vi "Measurements Add Items UI_Measure-Scope SP.vi"() -> ()   [LabVIEW 2012]
uses:
  Measurement Add Itmes Operations_Mesa.ctl
  <vilib>/Utility/miscctls.llb/LVPositionTypeDef.ctl
  Measure Operations_Meas.ctl
  Data Structure.llb/Function Variable Parameter Operations-Scope SP.ctl
  Data Structure.llb/Sub Panel Status Flag_DStr-Scope SP.vi
panel:
  out "Tab":enum32{"Volt", "Percent"}(tab)
  in  "Level":cluster{"High":dbl, "Mid":dbl, "Low":dbl} {"Low" min=-20.0 max=20.0 step=0.01 scale=-20.0..20.0; "Mid" min=-20.0 max=20.0 step=0.01 scale=-20.0..20.0 scale format="%#.2g"; "High" min=-20.0 max=20.0 step=0.01 scale=-20.0..20.0 scale format="%#.2f"}
  in  "Perc":cluster{"High":dbl, "Mid":dbl, "Low":dbl} {"Low" min=0.0 max=100.0 step=0.01 scale=0.0..100.0; "Mid" min=0.0 max=100.0 step=0.01 scale=0.0..100.0 scale format="%#.2g"; "High" min=0.0 max=100.0 step=0.01 scale=0.0..100.0 scale format="%#.2f"}
  in  "Config":T1
  in  "Temp":T3={"message"=variant, "measure"=refnum, "error"={"status"=FALSE, "code"=0, "source"=""}, "LevelRange"={"Max"=0.0, "Min"=0.0}, "Para"=1, "Percent"={"High"=0.0, "Mid"=0.0, "Low"=0.0}, "Level"={"High"=0.0, "Mid"=0.0, "Low"=0.0}}
  in  "Percent":i32(ring)=2 caption="百分比方式" items=["高低", "大小", "谷峰"]
  in  "Unit":i32(ring)=1 caption="单位" items=["伏特", "百分比"]
  in  "Help":bool
  in  "More...":bool
  in  "Cancel":bool
  in  "OK":bool
  in  "OtherChan":i32(ring) caption="其他通道" items=["0", "1"]
  in  "ParaSelec":i32(ring)=1 caption="测量参数" items=["设置参考电平", "频率", "平均频率", "FFT 频率", "周期", "平均周期", "上升时间", "下降时间", "上升压摆率", "下降压摆率", "过冲量", "预冲", "电压均方根", "电压周期均方根", "交流估计", "FFT幅值", "电压均值", "电压周期均值 ", "直流估计", "电压最大值", "电压最小值", "电压峰峰值", "电压高值", "电压低值 ", "电压幅值", "电压极点", "电压谷点", "电压最大差点", "负带宽", "正带宽", "负占空比", "正占空比", "积分", "面积", "周期面积", "延时", "相位延时", "低参考电压", "中参考电压", "高参考电压"]
  in  "Chan":i32(ring) caption="选择通道" items=["0", "1"]
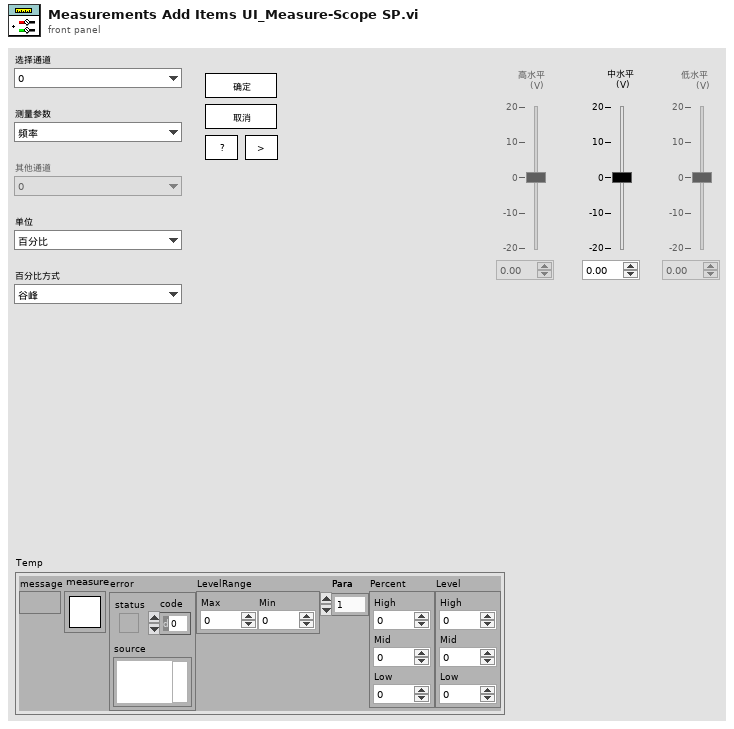
[diagram p1: front panel]
types:
  T1 = cluster{"Chan0":i32, "Para":string, "Chan1":i32, "Unit":i32, "Percent":i32, "High":dbl, "Mid":dbl, "Low":dbl, "ParaIndex":i32}
  T2 = typedef "Queue RefNum" = refnum<k1>
  T3 = cluster{"message":variant, "measure":T2, "error":errorcluster, "LevelRange":cluster{"Max":dbl, "Min":dbl}, "Para":i32, "Percent":cluster{"High":dbl, "Mid":dbl, "Low":dbl}, "Level":cluster{"High":dbl, "Mid":dbl, "Low":dbl}}
  T4 = typedef "Measurement Add Itmes Operations_Mesa.ctl" = enum16{"Initialize", "Initialize FP", "Idle", "Refresh FP", "ErrorHandle", "Close", "Exit"}
  T5 = typedef "LVPositionTypeDef.ctl" = cluster{"Left":i32, "Top":i32}
  T6 = typedef "LVRectTypeDef.ctl" = cluster{"Left":i16, "Top":i16, "Right":i16, "Bottom":i16}
  T7 = typedef "Function Variable Parameter Operations-Scope SP.ctl" = enum16{"Set", "Get"}
  T8 = typedef "Measure Operations_Meas.ctl" = enum16{"Add", "Config&Read", "Delete", "Clear"}
  T9 = cluster{"Para.":cluster{"Chans":cluster{"String":string, "Value":ext}[], "LevelRange":cluster{"Max":dbl, "Min":dbl}, "InstruHandle":refnum<k15>}, "Value":cluster{"Chan0":i32, "Para":string, "Chan1":i32, "Unit":i32, "Percent":i32, "High":dbl, "Mid":dbl, "Low":dbl, "ParaIndex":i32}[]}
  T10 = typedef "System Paths_FS-Scope SP.ctl" = cluster{"DeviceInfo":path, "SystemConstant":path, "INIDir":path}
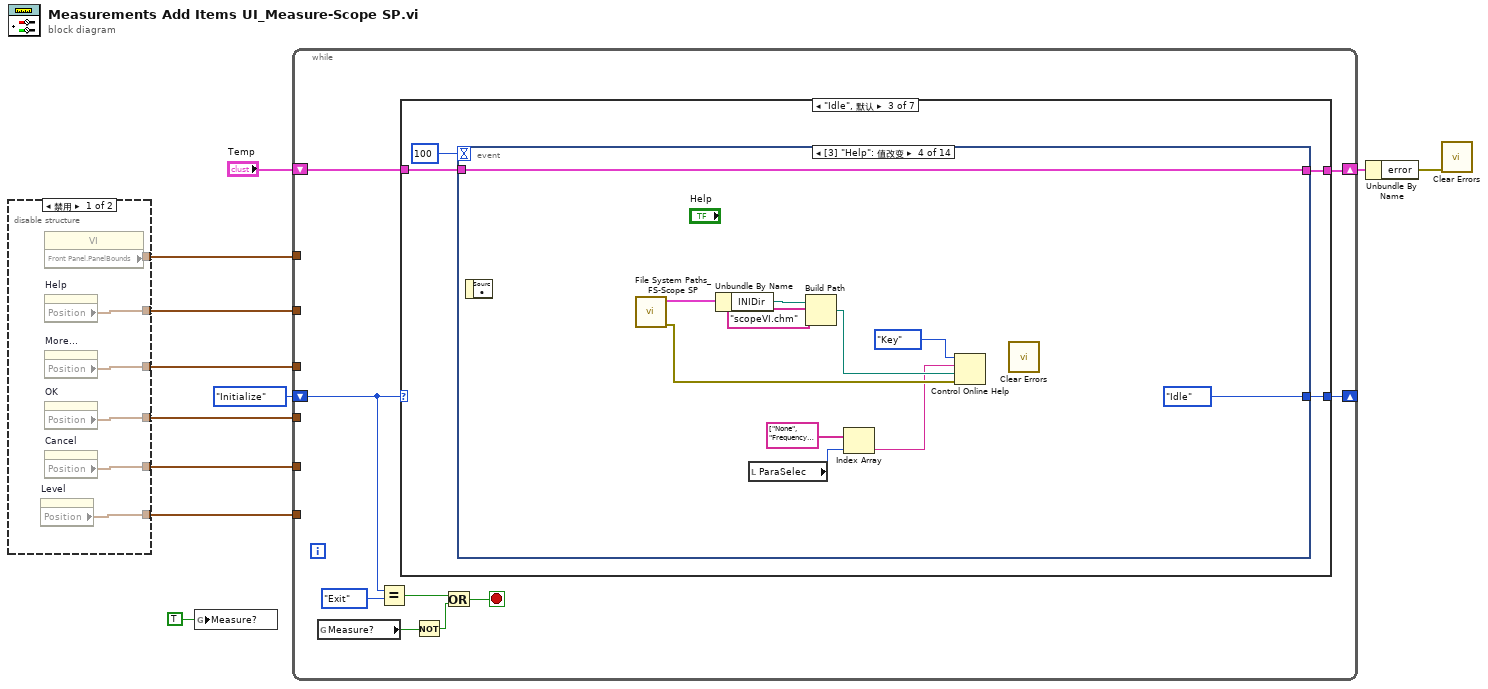
[diagram p0: block diagram]
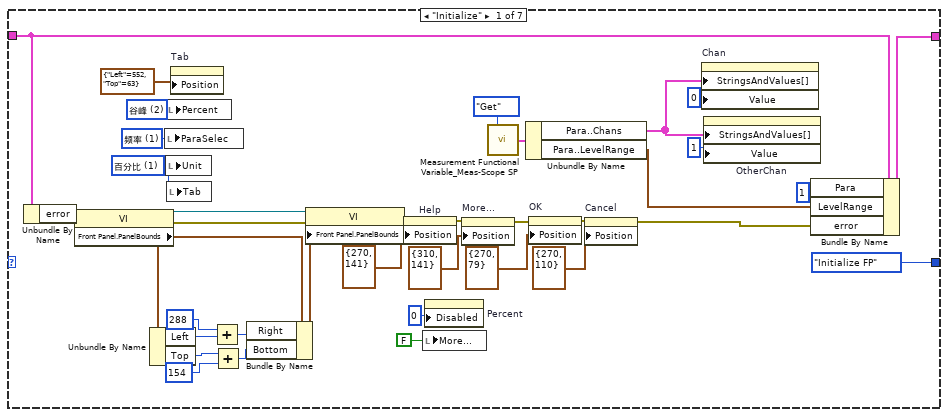
[diagram p3: hidden frame]
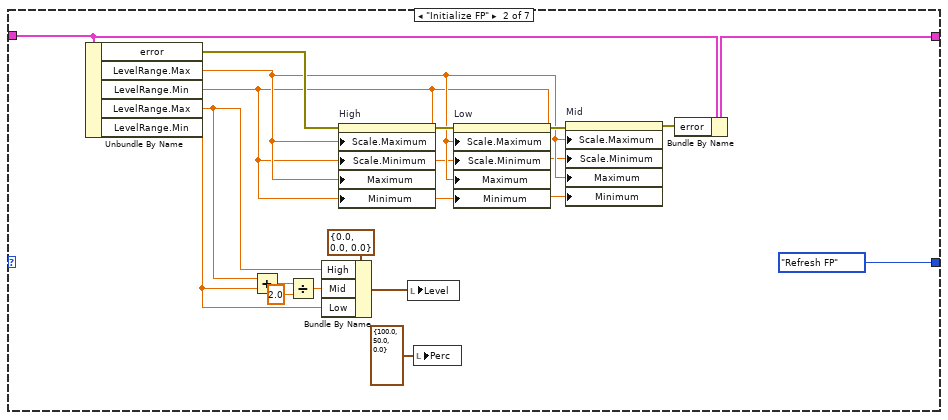
[diagram p4: hidden frame]
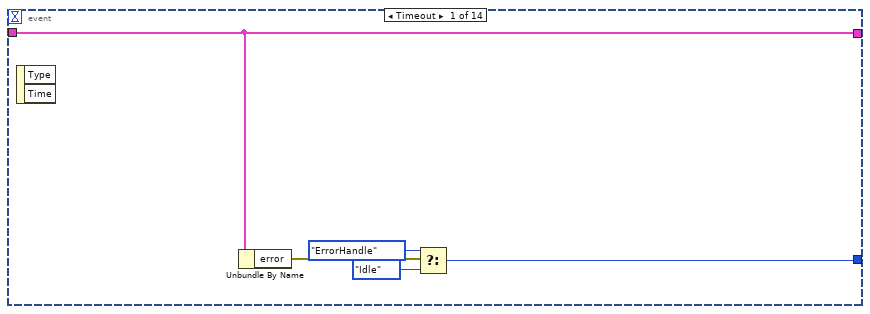
[diagram p5: hidden frame]
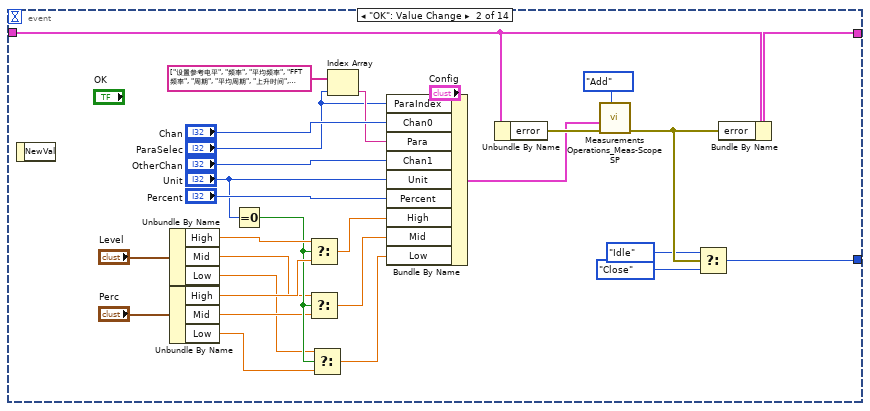
[diagram p6: hidden frame]
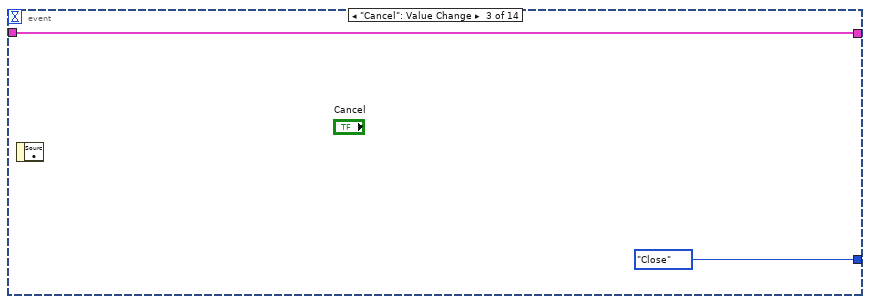
[diagram p7: hidden frame]
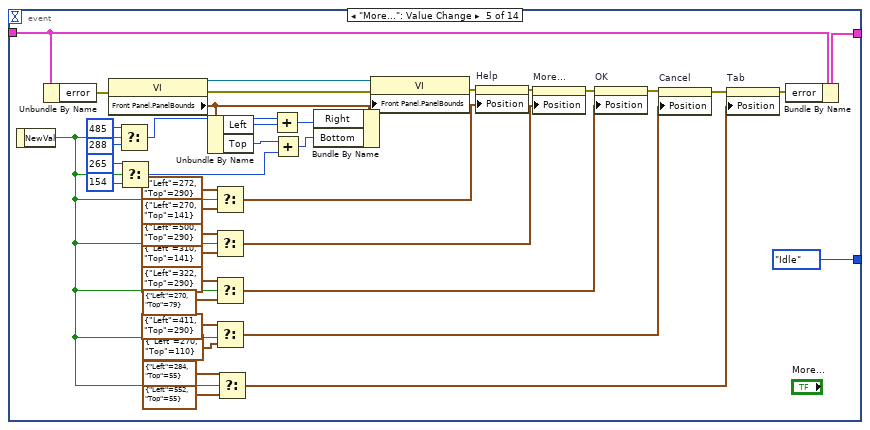
[diagram p8: hidden frame]
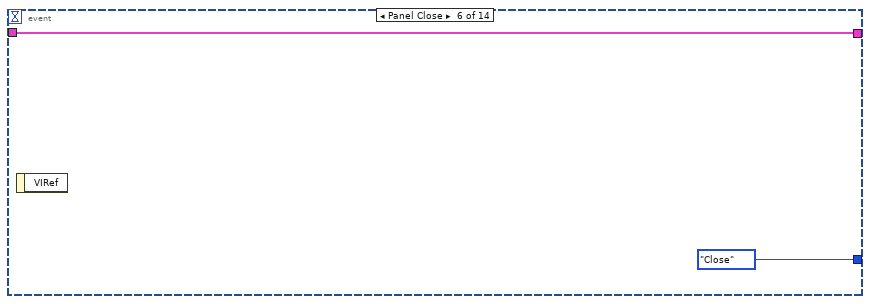
[diagram p9: hidden frame]
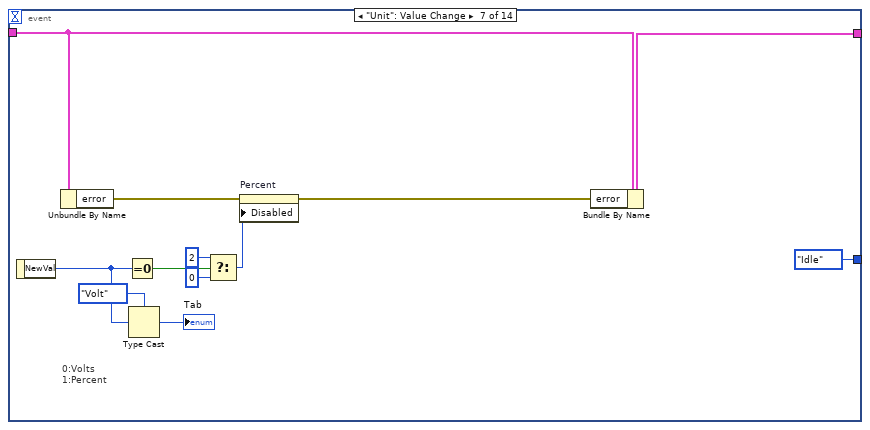
[diagram p10: hidden frame]
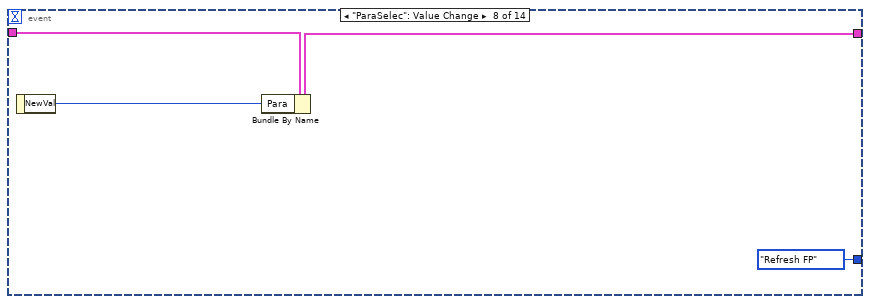
[diagram p11: hidden frame]
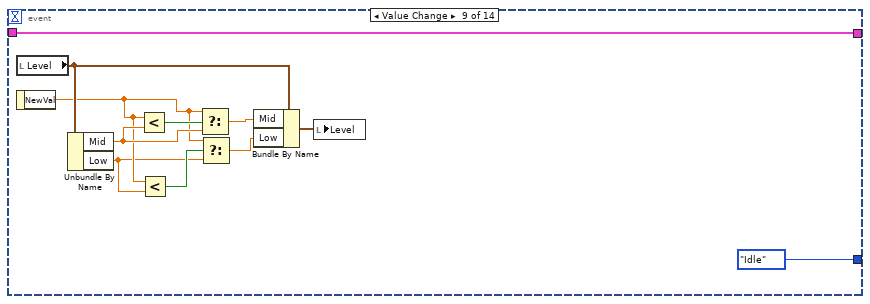
[diagram p12: hidden frame]
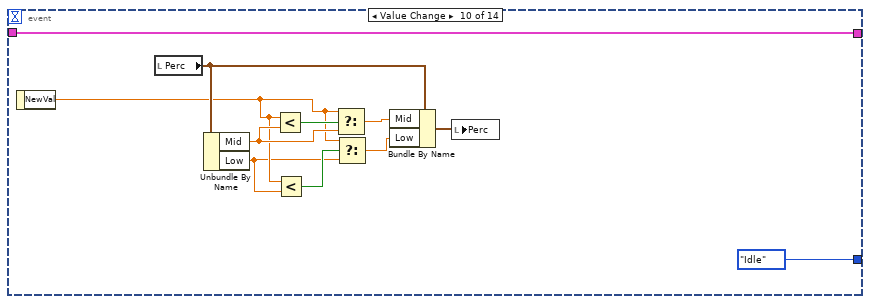
[diagram p13: hidden frame]
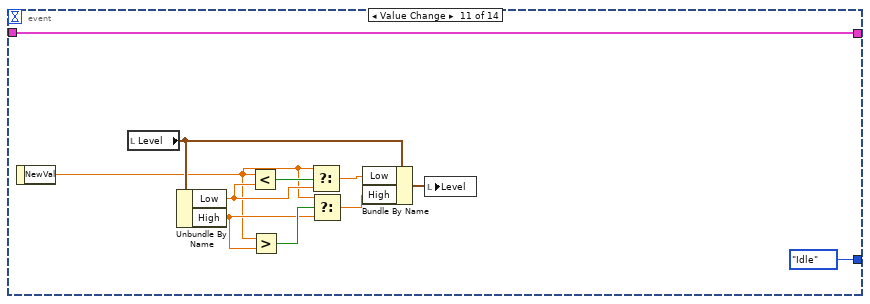
[diagram p14: hidden frame]
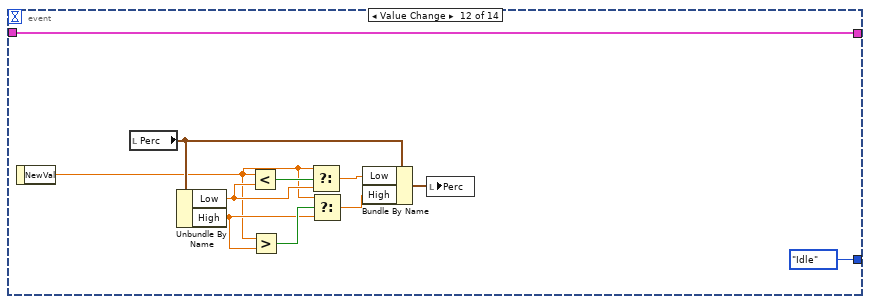
[diagram p15: hidden frame]
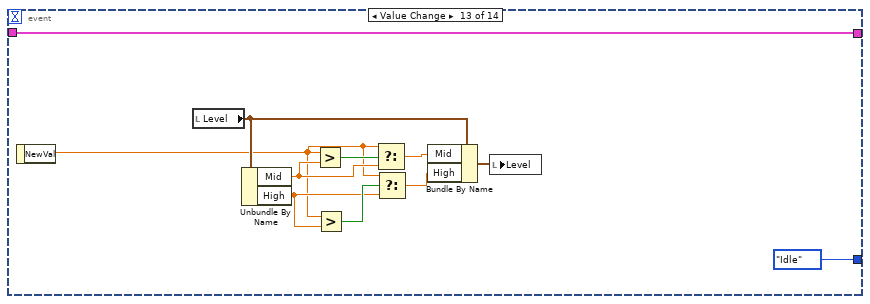
[diagram p16: hidden frame]
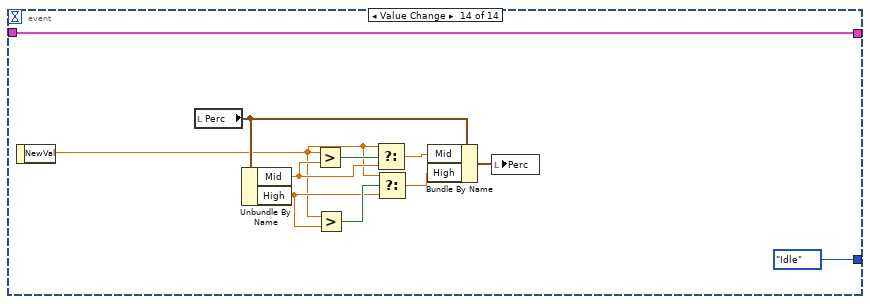
[diagram p17: hidden frame]
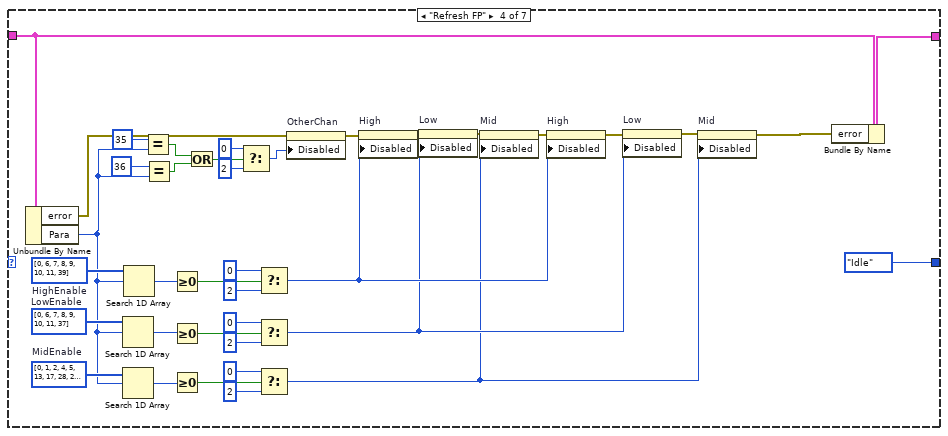
[diagram p18: hidden frame]
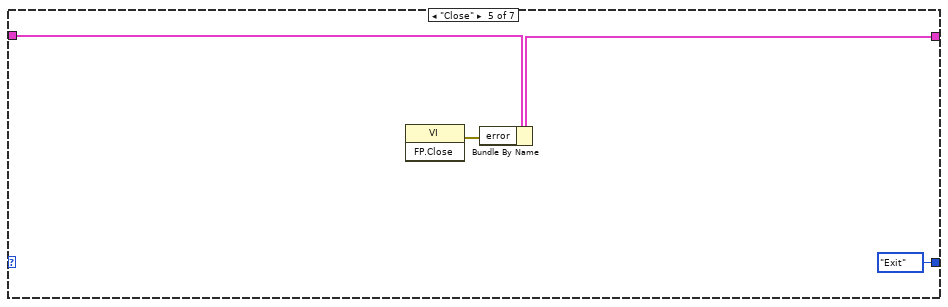
[diagram p19: hidden frame]
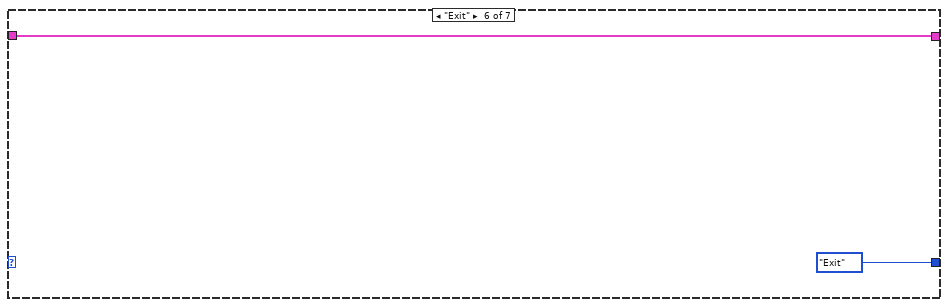
[diagram p20: hidden frame]
diagram:
  n1 = disable-structure shown="禁用" {
    disable-tunnel: [w17 _] -> w9
    disable-tunnel: [w16 _] -> w8
    disable-tunnel: [w15 _] -> w7
    disable-tunnel: [w14 _] -> w6
    disable-tunnel: [w13 _] -> w5
    disable-tunnel: [w12 _] -> w4
    frame Disabled {
      n2 = property on="Level" class="Clust (严格)"() -> ("Position"=w12:T5)  [unwired: 2 in, 2 out]
      n3 = property class="VI"() -> ("Front Panel.PanelBounds"=w13:T6)  [unwired: 2 in, 2 out]
      n4 = property on="Help" class="Bool"() -> ("Position"=w17:T5)  [unwired: 2 in, 2 out]
      n5 = property on="More..." class="Bool (严格)"() -> ("Position"=w16:T5)  [unwired: 2 in, 2 out]
      n6 = property on="OK" class="Bool"() -> ("Position"=w15:T5)  [unwired: 2 in, 2 out]
      n7 = property on="Cancel" class="Bool"() -> ("Position"=w14:T5)  [unwired: 2 in, 2 out]
    }
    frame Enabled {
    }
  }
  n8 = global write "Sub Panel Status Flag_DStr-Scope SP.vi" "Measure?"(TRUE ("Measure?")) -> ()
  n9 = while {
    shift-right: [w23] -> _
    shift-left: Measurement_Add_Itmes_Operations_Mesa."Initialize" ("Operations") -> [w25]
    shift-right: [w21] -> w2
    shift-left: "Temp" -> [w22]
    tunnel: w9 -> [_]
    tunnel: w8 -> [_]
    tunnel: w7 -> [_]
    tunnel: w6 -> [_]
    tunnel: w5 -> [_]
    tunnel: w4 -> [_]
    stop <- w20 stop-if-true
    n10 = global read "Sub Panel Status Flag_DStr-Scope SP.vi" "Measure?"() -> (w18:bool)
    n11 = Equal?(x=w25, y=Measurement_Add_Itmes_Operations_Mesa."Exit") -> (x = y?=w26:bool)
    n12 = case shown="\"Idle\", 默认" w25 {
      tunnel: [Measurement_Add_Itmes_Operations_Mesa."Initialize FP" ("Operations") Measurement_Add_Itmes_Operations_Mesa."Refresh FP" ("Operations") w82 Measurement_Add_Itmes_Operations_Mesa."Idle" ("Operations") Measurement_Add_Itmes_Operations_Mesa."Exit" ("Operations") Measurement_Add_Itmes_Operations_Mesa."Exit" ("Operations") Measurement_Add_Itmes_Operations_Mesa."Idle" ("Operations")] -> w23
      tunnel: w22 -> [w46 w72 w81 w275 w296 w297 w301]
      tunnel: [w45 w71 w80 w276 w294 w297 w300] -> w21
      frame "Initialize" {
        w37 = 2 items=["高低", "大小", "谷峰"] ("Percent")
        w34 = 1 items=["伏特", "百分比"] ("Unit")
        w38 = 1 items=["设置参考电平", "频率", "平均频率", "FFT 频率", "周期", "平均周期", "上升时间", "下降时间", "上升压摆率", "下降压摆率", "过冲量", "预冲", "电压均方根", "电压周期均方根", "交流估计", "FFT幅值", "电压均值", "电压周期均值 ", "直流估计", "电压最大值", "电压最小值", "电压峰峰值", "电压高值", "电压低值 ", "电压幅值", "电压极点", "电压谷点", "电压最大差点", "负带宽", "正带宽", "负占空比", "正占空比", "积分", "面积", "周期面积", "延时", "相位延时", "低参考电压", "中参考电压", "高参考电压"] ("Para")
        n13 = Unbundle By Name(w46) -> ("error"=w47:errorcluster)
        n14 = property class="VI"(error in=w47) -> (reference out=w60:refnum<vi>, error out=w61:errorcluster, "Front Panel.PanelBounds"=w55:T6)  [unwired: 1 in]
        n15 = Unbundle By Name(w55) -> ("Left"=w59:i16, "Top"=w58:i16)
        n16 = local write "ParaSelec"(w38) -> ()
        n17 = local write "Percent"(w37) -> ()
        n18 = local write "Unit"(w34) -> ()
        n19 = local write "Tab"(w34) -> ()
        n20 = property on="Tab" class="TabCtl (严格)"("Position"=T5 {"Left"=552, "Top"=63}) -> ()  [unwired: 2 in, 2 out]
        n21 = Add(x=i16 288, y=w59) -> (x+y=w54:i16)
        n22 = Add(x=w58, y=i16 154) -> (x+y=w53:i16)
        n23 = Bundle By Name(cluster=w55, "Right"=w54, "Bottom"=w53) -> (w52:T6)
        n24 = property class="VI"(reference=w60, error in=w61, "Front Panel.PanelBounds"=w52) -> (error out=w51:errorcluster)  [unwired: 1 out]
        n25 = property on="Help" class="Bool"(error in=w51, "Position"=T5 {"Left"=270, "Top"=141}) -> (error out=w50:errorcluster)  [unwired: 1 in, 1 out]
        n26 = local write "More..."(FALSE ("More...")) -> ()
        n27 = property on="Percent" class="Ring (严格)"("Disabled"=u8 0) -> ()  [unwired: 2 in, 2 out]
        n28 = property on="More..." class="Bool (严格)"(error in=w50, "Position"=T5 {"Left"=310, "Top"=141}) -> (error out=w44:errorcluster)  [unwired: 1 in, 1 out]
        n29 = call "Measurement Functional Variable_Meas-Scope SP.vi"("Mode(Get)"=Function_Variable_Parameter_Operations-Scope_SP."Get") -> ("MeasuConfig"=w31:T9)  [unwired: 14 in]
        n30 = Unbundle By Name(w31) -> ("Para..Chans"=w30:cluster{"String":string, "Value":ext}[], "Para..LevelRange"=w28:cluster{"Max":dbl, "Min":dbl})
        n31 = property on="OK" class="Bool"(error in=w44, "Position"=T5 {"Left"=270, "Top"=79}) -> (error out=w43:errorcluster)  [unwired: 1 in, 1 out]
        n32 = property on="Cancel" class="Bool"(error in=w43, "Position"=T5 {"Left"=270, "Top"=110}) -> (error out=w29:errorcluster)  [unwired: 1 in, 1 out]
        n33 = property on="Chan" class="Ring (严格)"("StringsAndValues[]"=w30, "Value"=0 ("OtherChan")) -> ()  [unwired: 2 in, 2 out]
        n34 = property on="OtherChan" class="Ring (严格)"("StringsAndValues[]"=w30, "Value"=1 ("OtherChan")) -> ()  [unwired: 2 in, 2 out]
        n35 = Bundle By Name(cluster=w46, "Para"=1, "LevelRange"=w28, "error"=w29) -> (w45:T3)
      }
      frame "Initialize FP" {
        n36 = Unbundle By Name(w72) -> ("error"=w76:errorcluster, "LevelRange.Max"=w75:dbl, "LevelRange.Min"=w74:dbl, "LevelRange.Max"=w68:dbl, "LevelRange.Min"=w67:dbl)
        n37 = Add(x=w68, y=w67) -> (x+y=w69:dbl)
        n38 = Divide(x=w69, y=2.0) -> (x/y=w66:dbl)
        n39 = Bundle By Name(cluster=cluster{"High":dbl, "Mid":dbl, "Low":dbl} {"High"=0.0, "Mid"=0.0, "Low"=0.0} ("Level"), "High"=w68, "Mid"=w66, "Low"=w67) -> (w64:cluster{"High":dbl, "Mid":dbl, "Low":dbl})
        n40 = property on="High" class="Slide (严格)"(error in=w76, "Scale.Maximum"=w75, "Scale.Minimum"=w74, "Maximum"=w75, "Minimum"=w74) -> (error out=w78:errorcluster)  [unwired: 1 in, 1 out]
        n41 = local write "Level"(w64) -> ()
        n42 = local write "Perc"(cluster{"High":dbl, "Mid":dbl, "Low":dbl} {"High"=100.0, "Mid"=50.0, "Low"=0.0} ("Perc")) -> ()
        n43 = property on="Low" class="Slide (严格)"(error in=w78, "Scale.Maximum"=w75, "Scale.Minimum"=w74, "Maximum"=w75, "Minimum"=w74) -> (error out=w77:errorcluster)  [unwired: 1 in, 1 out]
        n44 = property on="Mid" class="Slide (严格)"(error in=w77, "Scale.Maximum"=w75, "Scale.Minimum"=w74, "Maximum"=w75, "Minimum"=w74) -> (error out=w73:errorcluster)  [unwired: 1 in, 1 out]
        n45 = Bundle By Name(cluster=w72, "error"=w73) -> (w71:T3)
      }
      frame "Idle", Default {
        n46 = event shown="[3] \"Help\": 值改变" {
          selector: _ -> [_ _ _ _ _ _ _ _ _ _ _ _ _ _]
          dyn-events: _ -> [_ _ _ _ _ _ _ _ _ _ _ _ _ _]
          timeout: 100 -> [_ _ _ _ _ _ _ _ _ _ _ _ _ _]
          tunnel: [w84 w89 Measurement_Add_Itmes_Operations_Mesa."Close" ("Operations") Measurement_Add_Itmes_Operations_Mesa."Idle" ("Operations") Measurement_Add_Itmes_Operations_Mesa."Idle" ("Operations") Measurement_Add_Itmes_Operations_Mesa."Close" ("Operations") Measurement_Add_Itmes_Operations_Mesa."Idle" ("Operations") Measurement_Add_Itmes_Operations_Mesa."Refresh FP" ("Operations") Measurement_Add_Itmes_Operations_Mesa."Idle" ("Operations") Measurement_Add_Itmes_Operations_Mesa."Idle" ("Operations") Measurement_Add_Itmes_Operations_Mesa."Idle" ("Operations") Measurement_Add_Itmes_Operations_Mesa."Idle" ("Operations") Measurement_Add_Itmes_Operations_Mesa."Idle" ("Operations") Measurement_Add_Itmes_Operations_Mesa."Idle" ("Operations")] -> w82
          tunnel: w81 -> [w88 w100 w118 w129 w144 w172 w180 w188 w198 w209 w212 w223 w234 w245]
          tunnel: [w88 w99 w118 w129 w143 w172 w179 w186 w198 w209 w212 w223 w234 w245] -> w80
          event Timeout {
            n47 = event-data() -> ()  [unwired: 1 in, 2 out]
            n48 = Unbundle By Name(w88) -> ("error"=w87:errorcluster)
            n49 = Select(t=Measurement_Add_Itmes_Operations_Mesa."ErrorHandle" ("Operations"), s=w87, f=Measurement_Add_Itmes_Operations_Mesa."Idle" ("Operations")) -> (s? t:f=w84:T4)
          }
          event "OK": Value Change {
            n50 = event-data() -> ()  [unwired: 1 in, 1 out]
            n51 = Unbundle By Name("Level") -> ("High"=w110:dbl, "Mid"=w107:dbl, "Low"=w105:dbl)
            n52 = Unbundle By Name("Perc") -> ("High"=w109:dbl, "Mid"=w106:dbl, "Low"=w104:dbl)
            n53 = Equal To 0?(x="Unit") -> (x = 0?=w108:bool)
            n54 = Select(t=w110, s=w108, f=w109) -> (s? t:f=w103:dbl)
            n55 = Select(t=w107, s=w108, f=w106) -> (s? t:f=w102:dbl)
            n56 = Select(t=w105, s=w108, f=w104) -> (s? t:f=w101:dbl)
            n57 = Index Array(array=string[] ["设置参考电平", "频率", "平均频率", "FFT 频率", "周期", "平均周期", "上升时间", "下降时间", "上升压摆率", "下降压摆率", "过冲量", "预冲", "电压均方根", "电压周期均方根", "交流估计", "FFT幅值", "电压均值", "电压周期均值 ", "直流估计", "电压最大值", "电压最小值", "电压峰峰值", "电压高值", "电压低值 ", "电压幅值", "电压极点", "电压谷点", "电压最大差点", "负带宽", "正带宽", "负占空比", "正占空比", "积分", "面积", "周期面积", "延时", "相位延时", "低参考电压", "中参考电压", "高参考电压"] ("Para."), index="ParaSelec") -> (element=w97:string)
            n58 = Bundle By Name(cluster="Config", "ParaIndex"="ParaSelec", "Chan0"="Chan", "Para"=w97, "Chan1"="OtherChan", "Unit"="Unit", "Percent"="Percent", "High"=w103, "Mid"=w102, "Low"=w101) -> (w93:T1)
            n59 = Unbundle By Name(w100) -> ("error"=w95:errorcluster)
            n60 = call "Measurements Operations_Meas-Scope SP.vi"("Opearte"=Measure_Operations_Meas."Add", "error in"=w95, "Config"=w93) -> ("error out"=w92:errorcluster)  [unwired: 5 in, 3 out]
            n61 = Select(t=Measurement_Add_Itmes_Operations_Mesa."Idle" ("Operations"), s=w92, f=Measurement_Add_Itmes_Operations_Mesa."Close" ("Operations")) -> (s? t:f=w89:T4)
            n62 = Bundle By Name(cluster=w100, "error"=w92) -> (w99:T3)
          }
          event "Cancel": Value Change {
            n63 = event-data() -> ()  [unwired: 1 in, 1 out]
          }
          event "Help": Value Change {
            n64 = event-data() -> ()  [unwired: 1 in, 1 out]
            n65 = call "File System Paths_FS-Scope SP.vi"() -> ("error out"=w124:errorcluster, "FilePaths"=w125:T10)  [unwired: 9 in, 1 out]
            n66 = Unbundle By Name(w125) -> ("INIDir"=w127:path)
            n67 = local read "ParaSelec"() -> (w121:i32)
            n68 = Build Path(base path=w127, name or relative path="scopeVI.chm" ("名称或相对路径")) -> (appended path=w123:path)
            n69 = Index Array(array=string[] ["None", "Frequency", "Average Frequency", "FFT Frequency", "Period", "Average Period", "Rise Time", "Fall Time", "Rising Slew Rate", "Falling Slew Rate", "Overshoot", "Preshoot", "Voltage RMS", "Voltage Cycle RMS", "AC Estimate", "FFT Amplitude", "Voltage Average", "Voltage Cycle Average", "DC Estimate", "Voltage Max", "Voltage Min", "Voltage Peak-to-Peak", "Voltage High", "Voltage Low", "Voltage Amplitude", "Voltage Top", "Voltage Base", "Voltage Base-to-Top", "Negative Width", "Positive Width", "Negative Duty Cycle", "Positive Duty Cycle", "Integral", "Area", "Cycle Area", "Time Delay", "Phase Delay", "Low Ref Volts", "Mid Ref Volts", "High Ref Volts", "", "", "", "", "", "", "", "", "", "", "", "", "", "", "", "", "", "", "", "", "", "", "", ""] ("数组"), index=w121) -> (element=w120:string)
            n70 = Control Online Help(1:w124, 2:w123, 3:w120, 4:enum16{"Contents", "Key", "Close"}."Key" ("操作")) -> ()  [unwired: 1 out]
            n71 = call <vilib>:"Clear Errors.vi"() -> ()  [unwired: 7 in, 1 out]
          }
          event "More...": Value Change {
            n72 = event-data() -> ("NewVal"=w134:bool)  [unwired: 1 in]
            n73 = Unbundle By Name(w144) -> ("error"=w147:errorcluster)
            n74 = property class="VI"(error in=w147) -> (reference out=w169:refnum<vi>, error out=w170:errorcluster, "Front Panel.PanelBounds"=w166:T6)  [unwired: 1 in]
            n75 = Select(t=i16 485 ("x"), s=w134, f=i16 288 ("x")) -> (s? t:f=w158:i16)
            n76 = Select(t=i16 265 ("y"), s=w134, f=i16 154 ("y")) -> (s? t:f=w155:i16)
            n77 = Unbundle By Name(w166) -> ("Left"=w168:i16, "Top"=w167:i16)
            n78 = Select(t=T5 {"Left"=272, "Top"=290} ("Position"), s=w134, f=T5 {"Left"=270, "Top"=141} ("Position")) -> (s? t:f=w152:T5)
            n79 = Select(t=T5 {"Left"=500, "Top"=290} ("Position"), s=w134, f=T5 {"Left"=310, "Top"=141} ("Position")) -> (s? t:f=w149:T5)
            n80 = Select(t=T5 {"Left"=322, "Top"=290} ("Position"), s=w134, f=T5 {"Left"=270, "Top"=79} ("Position")) -> (s? t:f=w138:T5)
            n81 = Select(t=T5 {"Left"=411, "Top"=290} ("Position"), s=w134, f=T5 {"Left"=270, "Top"=110} ("Position")) -> (s? t:f=w137:T5)
            n82 = Select(t=T5 {"Left"=284, "Top"=55} ("Position"), s=w134, f=T5 {"Left"=552, "Top"=55} ("Position")) -> (s? t:f=w131:T5)
            n83 = Add(x=w158, y=w168) -> (x+y=w165:i16)
            n84 = Add(x=w167, y=w155) -> (x+y=w164:i16)
            n85 = Bundle By Name(cluster=w166, "Right"=w165, "Bottom"=w164) -> (w163:T6)
            n86 = property class="VI"(reference=w169, error in=w170, "Front Panel.PanelBounds"=w163) -> (error out=w162:errorcluster)  [unwired: 1 out]
            n87 = property on="Help" class="Bool"(error in=w162, "Position"=w152) -> (error out=w161:errorcluster)  [unwired: 1 in, 1 out]
            n88 = property on="More..." class="Bool (严格)"(error in=w161, "Position"=w149) -> (error out=w145:errorcluster)  [unwired: 1 in, 1 out]
            n89 = property on="OK" class="Bool"(error in=w145, "Position"=w138) -> (error out=w146:errorcluster)  [unwired: 1 in, 1 out]
            n90 = property on="Cancel" class="Bool"(error in=w146, "Position"=w137) -> (error out=w136:errorcluster)  [unwired: 1 in, 1 out]
            n91 = property on="Tab" class="TabCtl (严格)"(error in=w136, "Position"=w131) -> (error out=w135:errorcluster)  [unwired: 1 in, 1 out]
            n92 = Bundle By Name(cluster=w144, "error"=w135) -> (w143:T3)
          }
          event Panel Close {
            n93 = event-data() -> ()  [unwired: 1 in, 1 out]
          }
          event "Unit": Value Change {
            # "0:Volts\n1:Percent"
            n94 = event-data() -> ("NewVal"=w175:i32)  [unwired: 1 in]
            n95 = Unbundle By Name(w180) -> ("error"=w181:errorcluster)
            n96 = Equal To 0?(x=w175) -> (x = 0?=w178:bool)
            n97 = Type Cast(type=enum32{"Volt", "Percent"}."Volt" ("Tab"), x=w175) -> (*(type *) &x=→"Tab":enum32{"Volt", "Percent"})
            n98 = Select(t=u8 2 ("Disabled"), s=w178, f=u8 0 ("Disabled")) -> (s? t:f=w182:u8)
            n99 = property on="Percent" class="Ring (严格)"(error in=w181, "Disabled"=w182) -> (error out=w176:errorcluster)  [unwired: 1 in, 1 out]
            n100 = Bundle By Name(cluster=w180, "error"=w176) -> (w179:T3)
          }
          event "ParaSelec": Value Change {
            n101 = event-data() -> ("NewVal"=w187:i32)  [unwired: 1 in]
            n102 = Bundle By Name(cluster=w188, "Para"=w187) -> (w186:T3)
          }
          event "Level.High": Value Change {
            n103 = local read "Level"() -> (w197:cluster{"High":dbl, "Mid":dbl, "Low":dbl})
            n104 = event-data() -> ("NewVal"=w192:dbl)  [unwired: 1 in]
            n105 = Unbundle By Name(w197) -> ("Mid"=w195:dbl, "Low"=w190:dbl)
            n106 = Less?(x=w192, y=w195) -> (x < y?=w196:bool)
            n107 = Less?(x=w192, y=w190) -> (x < y?=w193:bool)
            n108 = Select(t=w192, s=w196, f=w195) -> (s? t:f=w194:dbl)
            n109 = Select(t=w192, s=w193, f=w190) -> (s? t:f=w191:dbl)
            n110 = Bundle By Name(cluster=w197, "Mid"=w194, "Low"=w191) -> (w189:cluster{"High":dbl, "Mid":dbl, "Low":dbl})
            n111 = local write "Level"(w189) -> ()
          }
          event "Perc.High": Value Change {
            n112 = event-data() -> ("NewVal"=w203:dbl)  [unwired: 1 in]
            n113 = local read "Perc"() -> (w208:cluster{"High":dbl, "Mid":dbl, "Low":dbl})
            n114 = Unbundle By Name(w208) -> ("Mid"=w206:dbl, "Low"=w201:dbl)
            n115 = Less?(x=w203, y=w206) -> (x < y?=w207:bool)
            n116 = Less?(x=w203, y=w201) -> (x < y?=w204:bool)
            n117 = Select(t=w203, s=w207, f=w206) -> (s? t:f=w205:dbl)
            n118 = Select(t=w203, s=w204, f=w201) -> (s? t:f=w202:dbl)
            n119 = Bundle By Name(cluster=w208, "Mid"=w205, "Low"=w202) -> (w200:cluster{"High":dbl, "Mid":dbl, "Low":dbl})
            n120 = local write "Perc"(w200) -> ()
          }
          event "Level.Mid": Value Change {
            n121 = event-data() -> ("NewVal"=w213:dbl)  [unwired: 1 in]
            n122 = local read "Level"() -> (w221:cluster{"High":dbl, "Mid":dbl, "Low":dbl})
            n123 = Unbundle By Name(w221) -> ("Low"=w219:dbl, "High"=w215:dbl)
            n124 = Less?(x=w213, y=w219) -> (x < y?=w220:bool)
            n125 = Greater?(x=w213, y=w215) -> (0:w217:bool)
            n126 = Select(t=w213, s=w220, f=w219) -> (s? t:f=w218:dbl)
            n127 = Select(t=w213, s=w217, f=w215) -> (s? t:f=w216:dbl)
            n128 = Bundle By Name(cluster=w221, "Low"=w218, "High"=w216) -> (w214:cluster{"High":dbl, "Mid":dbl, "Low":dbl})
            n129 = local write "Level"(w214) -> ()
          }
          event "Perc.Mid": Value Change {
            n130 = event-data() -> ("NewVal"=w224:dbl)  [unwired: 1 in]
            n131 = local read "Perc"() -> (w232:cluster{"High":dbl, "Mid":dbl, "Low":dbl})
            n132 = Unbundle By Name(w232) -> ("Low"=w230:dbl, "High"=w226:dbl)
            n133 = Less?(x=w224, y=w230) -> (x < y?=w231:bool)
            n134 = Greater?(x=w224, y=w226) -> (0:w228:bool)
            n135 = Select(t=w224, s=w231, f=w230) -> (s? t:f=w229:dbl)
            n136 = Select(t=w224, s=w228, f=w226) -> (s? t:f=w227:dbl)
            n137 = Bundle By Name(cluster=w232, "Low"=w229, "High"=w227) -> (w225:cluster{"High":dbl, "Mid":dbl, "Low":dbl})
            n138 = local write "Perc"(w225) -> ()
          }
          event "Level.Low": Value Change {
            n139 = event-data() -> ("NewVal"=w235:dbl)  [unwired: 1 in]
            n140 = local read "Level"() -> (w243:cluster{"High":dbl, "Mid":dbl, "Low":dbl})
            n141 = Unbundle By Name(w243) -> ("Mid"=w241:dbl, "High"=w237:dbl)
            n142 = Greater?(x=w235, y=w241) -> (0:w242:bool)
            n143 = Greater?(x=w235, y=w237) -> (0:w239:bool)
            n144 = Select(t=w235, s=w242, f=w241) -> (s? t:f=w240:dbl)
            n145 = Select(t=w235, s=w239, f=w237) -> (s? t:f=w238:dbl)
            n146 = Bundle By Name(cluster=w243, "Mid"=w240, "High"=w238) -> (w236:cluster{"High":dbl, "Mid":dbl, "Low":dbl})
            n147 = local write "Level"(w236) -> ()
          }
          event "Perc.Low": Value Change {
            n148 = event-data() -> ("NewVal"=w246:dbl)  [unwired: 1 in]
            n149 = local read "Perc"() -> (w254:cluster{"High":dbl, "Mid":dbl, "Low":dbl})
            n150 = Unbundle By Name(w254) -> ("Mid"=w252:dbl, "High"=w248:dbl)
            n151 = Greater?(x=w246, y=w252) -> (0:w253:bool)
            n152 = Greater?(x=w246, y=w248) -> (0:w250:bool)
            n153 = Select(t=w246, s=w253, f=w252) -> (s? t:f=w251:dbl)
            n154 = Select(t=w246, s=w250, f=w248) -> (s? t:f=w249:dbl)
            n155 = Bundle By Name(cluster=w254, "Mid"=w251, "High"=w249) -> (w247:cluster{"High":dbl, "Mid":dbl, "Low":dbl})
            n156 = local write "Perc"(w247) -> ()
          }
        }
      }
      frame "Refresh FP" {
        w271 = i32[] [0, 1, 2, 4, 5, 13, 17, 28, 29, 30, 31, 34, 35, 36, 38]  # MidEnable
        w272 = i32[] [0, 6, 7, 8, 9, 10, 11, 37]  # LowEnable
        w273 = i32[] [0, 6, 7, 8, 9, 10, 11, 39]  # HighEnable
        n157 = Unbundle By Name(w275) -> ("error"=w277:errorcluster, "Para"=w270:i32)
        n158 = Search 1D Array(1D array=w272, element=w270) -> (index of element=w268:i32)  [unwired: 1 in]
        n159 = Search 1D Array(1D array=w271, element=w270) -> (index of element=w267:i32)  [unwired: 1 in]
        n160 = Search 1D Array(1D array=w273, element=w270) -> (index of element=w269:i32)  [unwired: 1 in]
        n161 = Equal?(x=35, y=w270) -> (x = y?=w291:bool)
        n162 = Equal?(x=36, y=w270) -> (x = y?=w289:bool)
        n163 = Greater Or Equal To 0?(x=w269) -> (x >= 0?=w264:bool)
        n164 = Greater Or Equal To 0?(x=w268) -> (x >= 0?=w261:bool)
        n165 = Greater Or Equal To 0?(x=w267) -> (x >= 0?=w258:bool)
        n166 = Or(x=w291, y=w289) -> (x .or. y?=w288:bool)
        n167 = Select(t=u8 0 ("x"), s=w288, f=u8 2 ("x")) -> (s? t:f=w285:u8)
        n168 = Select(t=u8 0 ("x"), s=w264, f=u8 2 ("x")) -> (s? t:f=w257:u8)
        n169 = Select(t=u8 0 ("x"), s=w261, f=u8 2 ("x")) -> (s? t:f=w256:u8)
        n170 = Select(t=u8 0 ("x"), s=w258, f=u8 2 ("x")) -> (s? t:f=w255:u8)
        n171 = property on="OtherChan" class="Ring (严格)"(error in=w277, "Disabled"=w285) -> (error out=w284:errorcluster)  [unwired: 1 in, 1 out]
        n172 = property on="High" class="Slide (严格)"(error in=w284, "Disabled"=w257) -> (error out=w283:errorcluster)  [unwired: 1 in, 1 out]
        n173 = property on="Low" class="Slide (严格)"(error in=w283, "Disabled"=w256) -> (error out=w282:errorcluster)  [unwired: 1 in, 1 out]
        n174 = property on="Mid" class="Slide (严格)"(error in=w282, "Disabled"=w255) -> (error out=w281:errorcluster)  [unwired: 1 in, 1 out]
        n175 = property on="High" class="Slide (严格)"(error in=w281, "Disabled"=w257) -> (error out=w280:errorcluster)  [unwired: 1 in, 1 out]
        n176 = property on="Low" class="Slide (严格)"(error in=w280, "Disabled"=w256) -> (error out=w279:errorcluster)  [unwired: 1 in, 1 out]
        n177 = property on="Mid" class="Slide (严格)"(error in=w279, "Disabled"=w255) -> (error out=w274:errorcluster)  [unwired: 1 in, 1 out]
        n178 = Bundle By Name(cluster=w275, "error"=w274) -> (w276:T3)
      }
      frame "Close" {
        n179 = invoke class="VI" method="FP.Close"() -> (error out=w295:errorcluster)  [unwired: 3 in, 2 out]
        n180 = Bundle By Name(cluster=w296, "error"=w295) -> (w294:T3)
      }
      frame "Exit" {
      }
      frame "ErrorHandle" {
        n181 = Unbundle By Name(w301) -> ("error"=w304:errorcluster)
        n182 = call <vilib>:"Simple Error Handler.vi"("error in (no error)"=w304) -> ("error out"=w303:errorcluster)  [unwired: 4 in, 4 out]
        n183 = call "Error Clear Errors__Uti.vi"("error in (no error)"=w303) -> ("error out"=w302:errorcluster)  [unwired: 6 in]
        n184 = Bundle By Name(cluster=w301, "error"=w302) -> (w300:T3)
      }
    }
    n185 = Not(x=w18) -> (.not. x?=w19:bool)
    n186 = Or(x=w26, y=w19) -> (x .or. y?=w20:bool)
  }
  n187 = Unbundle By Name(w2) -> ("error"=w1:errorcluster)
  n188 = call <vilib>:"Clear Errors.vi"("error in (no error)"=w1) -> ()  [unwired: 6 in, 1 out]
